vi "DIOSerialPortRx.vi"(11 "DIOSerialPortSettings":T1={"TxPort"="ModbusPort1Tx", "TxDataFIFO"="ModbusPort1TxFIFO", "RxPort"="ModbusPort1Rx", "RxDataFIFO"="ModbusPort1RxFIFO"}) -> ()   [LabVIEW 2016]
uses:
  DIOSerialPortSettings.ctl
  DIOSerialPortRxData.ctl
  DIOSerialPortRxStates.ctl
  <vilib>/Platform/TimedLoop/XDataNode/timing_clust.ctl
  <vilib>/Platform/TimedLoop/XDataNode/nitl_modes.ctl
  <vilib>/Platform/TimedLoop/XDataNode/wakeup.ctl
  <vilib>/rvi/Emulation/niFpgaSctlEmulationGetInTimedLoop.vi
  <vilib>/rvi/Emulation/niFpgaEmulationReportErrorSimple.vi
  <vilib>/rvi/Emulation/niFpgaGetClockAttributes.vi
  <vilib>/rvi/Emulation/niFpgaCriticalErrorInLSC.vi
  <vilib>/rvi/eio/common/nirviEmuTemplateMethod_errors.vi
  <vilib>/rvi/DataTransferAndStorage/Container/Common/niFpgaContainerExecOnDevCompGetState.vi
  <vilib>/rvi/Emulation/niFpgaEmulationIsFPGAContextNoSignature.vi
  <vilib>/rvi/errors/niFpgaSetErrorForExecOnDevCompSimple.vi
  <vilib>/rvi/eio/common/nirviEmuReportErrorAndStop.vi
  <vilib>/rvi/DataTransferAndStorage/Container/Common/niFpgaContainerGetUniqueNameForEmu.vi
  <vilib>/rvi/FIFO/Fifo_Resource/nirvififoEmulationSetSize.vi
  <vilib>/rvi/FIFO/Fifo_Resource/nirviFifoEmulationQueueMgr.vi
  <instcachedir>/0/nirviFifoEmulationQueueMgr_E5CAEC123FF24DC58D834DCA3CDAA9B5.lvgen/nirviFifoEmulationQueueMgr_E5CAEC123FF24DC58D834DCA3CDAA9B5_009.vi
  <vilib>/rvi/FIFO/Fifo_Resource/nirvififoEmulationDetermineInputValidOut.vi
  <vilib>/rvi/FIFO/Fifo_Resource/nirvififoEmulationCreateLock.vi
  <vilib>/rvi/Emulation/niFpgaProcessEmulError.vi
  <vilib>/rvi/FIFO/Fifo_Resource/nirvififoEmulationObtainLock.vi
  <vilib>/rvi/FIFO/Fifo_Resource/nirvififoEmulationReleaseLock.vi
  <vilib>/rvi/occurrence/nirviWaitOnOccurrenceBase.vi
  <vilib>/rvi/errors/nirviReportUnexpectedCaseInternalError.vi
  <vilib>/rvi/errors/nirviReportUnexpectedCaseInternalError (U32).vi
  <vilib>/Utility/error.llb/Clear Errors.vi
  <vilib>/rvi/interface/RandomDataEmulation/niFpgaRandomDataHandleErrors.vi
  <vilib>/Platform/TimedLoop/XDataNode/XDataNode.xnode
  <vilib>/eio/EIONode/EIONode.xnode
  <vilib>/rvi/DataTransferAndStorage/Container/XNode/niFpgaContainer.xnode
  <vilib>/rvi/FIFO/Fifo_Resource/niFpgaFifoEmulationRefIn.vi
  <vilib>/Platform/TimedLoop/XDataNode/XDNodeRunTimeDep.lvlib
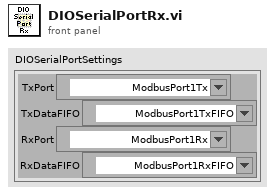
[diagram p1: front panel]
types:
  T1 = typedef "DIOSerialPortSettings.ctl" = cluster{"TxPort":refnum<k21>, "TxDataFIFO":refnum<k21>, "RxPort":refnum<k21>, "RxDataFIFO":refnum<k21>}
  T2 = typedef "DIOSerialPortRxData.ctl" = cluster{"State":T3, "DelayTicks":u8, "StateAfterDelay":T3, "Data":u8, "Bit":u8, "StartBit":u8, "StopBit":u8, "PreviousState":bool}
  T3 = typedef "DIOSerialPortRxStates.ctl" = enum16{"WaitForFallingEdge", "SampleStartBit", "SampleDataBits", "SampleStopBit", "Delay", "EnqueueData"}
  T4 = typedef "XDNodeRunTimeDep.lvlib/timing_clust.ctl" = cluster{"Expected End [f-1]":u64, "Actual End [f-1]":u64, "Finished Late? [f-1]":bool, "Expected End [i-1]":u64, "Actual End [i-1]":u64, "Finished Late? [i-1]":bool, "Expected Start [i]":u64, "Actual Start [i]":u64, "Expected Start [f]":u64, "Actual Start [f]":u64, "Source Name":string, "Structure Name":string, "Period":i64, "Deadline":i64, "Offset":i64, "Start":i64, "Priority":i32, "Timeout":i32, "Mode":T5, "Wakeup Reason":T6, "Error":errorcluster, "Source Type":string, "Secondary Source Type":string, "Global End Time":u64, "Global Start Time":u64, "Frame Duration":u64, "Iteration Duration":u64, "Assigned CPU":i32, "I/O Scan Engine Mode":u32}
  T5 = typedef "XDNodeRunTimeDep.lvlib/nitl_modes.ctl" = enum32{"No Change", "Process missed periods, maintain original phase", "Discard missed periods, maintain original phase", "Process missed periods, ignore original phase", "Discard missed periods, ignore original phase"}
  T6 = typedef "XDNodeRunTimeDep.lvlib/wakeup.ctl" = enum32{"Normal", "Aborted", "Asynchronous wakeup", "Timing source error", "Timed loop error", "Timeout"}
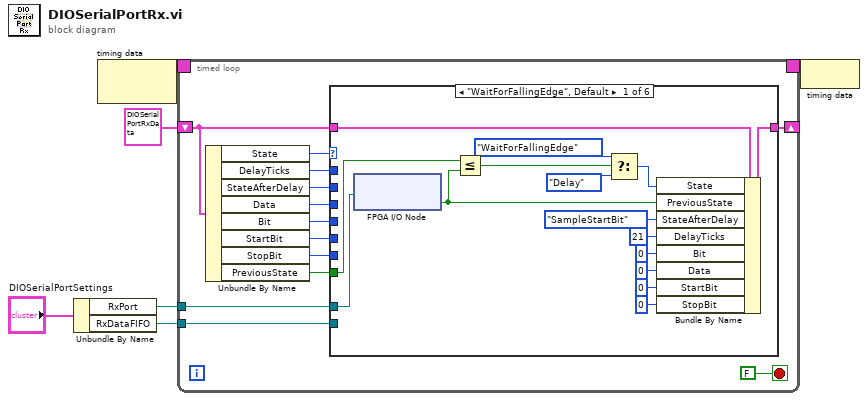
[diagram p0: block diagram]
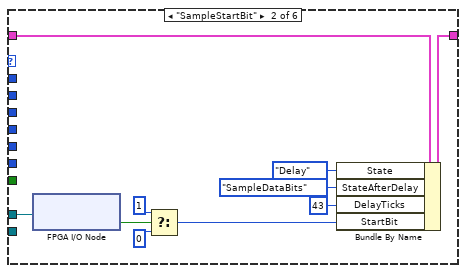
[diagram p2: hidden frame]
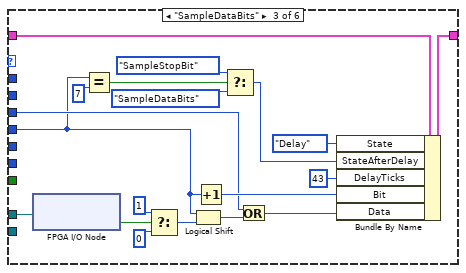
[diagram p3: hidden frame]
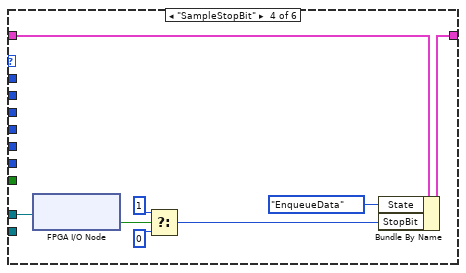
[diagram p4: hidden frame]
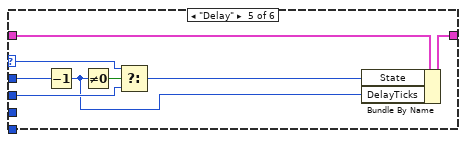
[diagram p5: hidden frame]
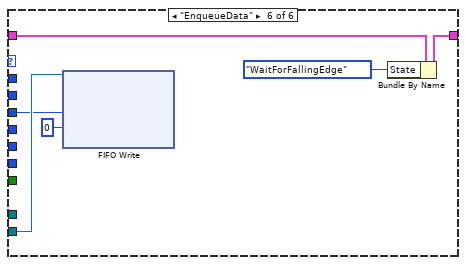
[diagram p6: hidden frame]
diagram:
  n1 = Unbundle By Name("DIOSerialPortSettings") -> ("RxPort"=w2:refnum<k21>, "RxDataFIFO"=w1:refnum<k21>)
  n2 = node-c288() -> (w6:T4)  [unwired: 1 in]
  n3 = timed-loop {
    timing: w6 -> [_]
    timing-out: [_] -> w5
    shift-right: [w15] -> _
    shift-left: T2 {"State"=enum."WaitForFallingEdge", "DelayTicks"=0, "StateAfterDelay"=enum."WaitForFallingEdge", "Data"=0, "Bit"=0, "StartBit"=0, "StopBit"=0, "PreviousState"=FALSE} ("DIOSerialPortRxData") -> [w19]
    tunnel: w2 -> [w17]
    tunnel: w1 -> [w8]
    stop <- FALSE stop-if-true
    n4 = Unbundle By Name(w19) -> ("State"=w18:T3, "DelayTicks"=w9:u8, "StateAfterDelay"=w10:T3, "Data"=w11:u8, "Bit"=w14:u8, "StartBit"=w13:u8, "StopBit"=w12:u8, "PreviousState"=w16:bool)
    n5 = case shown="\"WaitForFallingEdge\", Default" w18 {
      selector: w18 -> [_ _ _ _ w75 _]
      tunnel: w19 -> [w29 w43 w62 w70 w79 w85]
      tunnel: w17 -> [w34 w44 w63 w71 _ _]
      tunnel: w16 -> [w33 _ _ _ _ _]
      tunnel: [w28 w42 w61 w69 w78 w84] -> w15
      tunnel: w14 -> [_ _ w50 _ _ _]
      tunnel: w13 -> [_ _ _ _ _ _]
      tunnel: w12 -> [_ _ _ _ _ _]
      tunnel: w11 -> [_ _ w52 _ _ w81]
      tunnel: w10 -> [_ _ _ _ w74 _]
      tunnel: w9 -> [_ _ _ _ w76 _]
      tunnel: w8 -> [_ _ _ _ _ w82]
      frame "WaitForFallingEdge", Default {
        n6 = xnode "FPGA I/O Node"("FPGA I/O In"=w34) -> ("I/O Item"=w26:bool)  [unwired: 1 out]
        n7 = Less Or Equal?(x=w33, y=w26) -> (x <= y?=w32:bool)
        n8 = Select(t=DIOSerialPortRxStates."WaitForFallingEdge" ("DIOSerialPortRxStates"), s=w32, f=DIOSerialPortRxStates."Delay" ("DIOSerialPortRxStates")) -> (s? t:f=w27:T3)
        n9 = Bundle By Name(cluster=w29, "State"=w27, "PreviousState"=w26, "StateAfterDelay"=DIOSerialPortRxStates."SampleStartBit", "DelayTicks"=u8 21, "Bit"=u8 0, "Data"=u8 0, "StartBit"=u8 0, "StopBit"=u8 0) -> (w28:T2)
      }
      frame "SampleStartBit" {
        n10 = xnode "FPGA I/O Node"("FPGA I/O In"=w44) -> ("I/O Item"=w40:bool)  [unwired: 1 out]
        n11 = Select(t=u8 1, s=w40, f=u8 0) -> (s? t:f=w35:u8)
        n12 = Bundle By Name(cluster=w43, "State"=DIOSerialPortRxStates."Delay" ("StateAfterDelay"), "StateAfterDelay"=DIOSerialPortRxStates."SampleDataBits", "DelayTicks"=u8 43, "StartBit"=w35) -> (w42:T2)
      }
      frame "SampleDataBits" {
        n13 = xnode "FPGA I/O Node"("FPGA I/O In"=w63) -> ("I/O Item"=w59:bool)  [unwired: 1 out]
        n14 = Equal?(x=w50, y=u8 7) -> (x = y?=w48:bool)
        n15 = Select(t=u8 1, s=w59, f=u8 0) -> (s? t:f=w55:u8)
        n16 = Logical Shift(y=w50, x=w55) -> (x << y=w53:u8)
        n17 = Increment(x=w50) -> (x+1=w54:u8)
        n18 = Select(t=DIOSerialPortRxStates."SampleStopBit" ("StateAfterDelay"), s=w48, f=DIOSerialPortRxStates."SampleDataBits" ("StateAfterDelay")) -> (s? t:f=w45:T3)
        n19 = Or(x=w52, y=w53) -> (x .or. y?=w51:u8)
        n20 = Bundle By Name(cluster=w62, "State"=DIOSerialPortRxStates."Delay" ("StateAfterDelay"), "StateAfterDelay"=w45, "DelayTicks"=u8 43, "Bit"=w54, "Data"=w51) -> (w61:T2)
      }
      frame "SampleStopBit" {
        n21 = xnode "FPGA I/O Node"("FPGA I/O In"=w71) -> ("I/O Item"=w68:bool)  [unwired: 1 out]
        n22 = Select(t=u8 1, s=w68, f=u8 0) -> (s? t:f=w64:u8)
        n23 = Bundle By Name(cluster=w70, "State"=DIOSerialPortRxStates."EnqueueData" ("StateAfterDelay"), "StopBit"=w64) -> (w69:T2)
      }
      frame "Delay" {
        n24 = Decrement(x=w76) -> (x-1=w72:u8)
        n25 = Not Equal To 0?(x=w72) -> (x != 0?=w77:bool)
        n26 = Select(t=w75, s=w77, f=w74) -> (s? t:f=w73:T3)
        n27 = Bundle By Name(cluster=w79, "State"=w73, "DelayTicks"=w72) -> (w78:T2)
      }
      frame "EnqueueData" {
        n28 = xnode ("FIFO Write")("Element"=w81, "Timeout"=0, "FIFO In"=w82) -> ()  [unwired: 2 out]
        n29 = Bundle By Name(cluster=w85, "State"=DIOSerialPortRxStates."WaitForFallingEdge") -> (w84:T2)
      }
    }
  }
  n30 = node-c288(w5) -> ()
